vi "energyFromWaveForm.vi"(11 "Array in":waveform(dbl)[](array[waveform])) -> (3 "results":dbl[](array[numeric]))   [LabVIEW 2013]
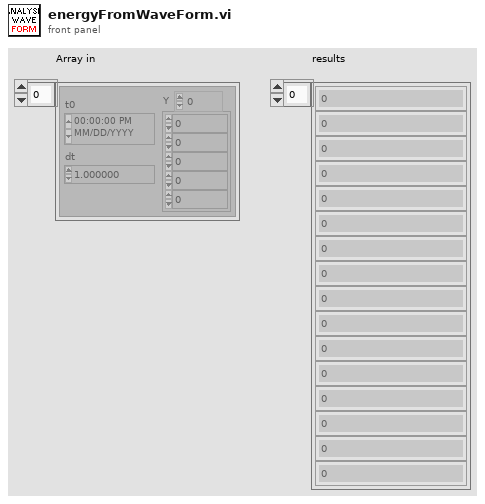
[diagram p1: front panel]
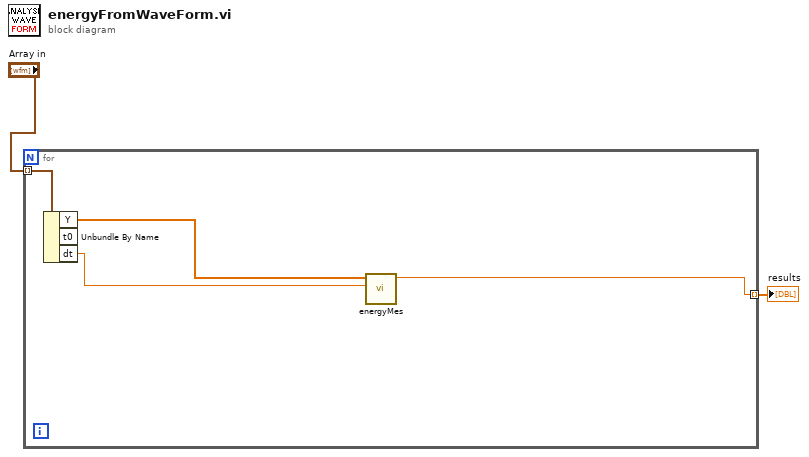
[diagram p0: block diagram]
diagram:
  n1 = for {
    tunnel: "Array in" -> [w6] mode=indexing
    tunnel: [w3] -> w2 mode=indexing
    n2 = Unbundle By Name(w6) -> ("Y"=w5:dbl[], "dt"=w4:dbl)  [unwired: 1 out]
    n3 = call "energyMes.vi"("dt"=w4, "Y"=w5) -> ("result"=w3:dbl)  [unwired: 9 in]
  }
  "results" <- w2
